vi "TruncI64.vi"(5 "Decimal places":i8, 6 "Number":i64) -> (2 "Truncated number":i64)   [LabVIEW 2017, in "GPNumeric.lvlib"]
doc: "Truncates <B>Number</B> to a number of <B>Decimal places</B>.\n\nSet <B>Decimal places</B> to a negative number to truncate to nearest 10, nearest 100 and so on. E.g. to truncate 782 to the nearest hundred, you set <B>Decimal places</B> to -2 and the <B>Truncated number</B> will be 700.\n\nThis VI is inlined.\n\nSteen Schmidt\nGPower\n16/5 2014"
uses:
  GPNumeric.lvlib
panel:
  # "Copyright © 2014\nGPower\nSee enclosed license file for terms and conditions"
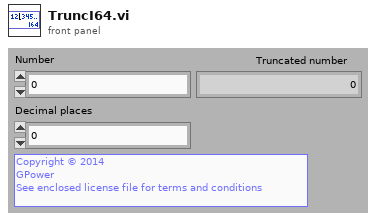
[diagram p1: front panel]
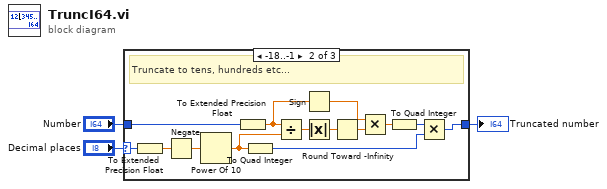
[diagram p0: block diagram]
diagram:
  n1 = case shown="-18..-1" "Decimal places" {
    selector: "Decimal places" -> [_ w14 _]
    tunnel: [_ w11 w18] -> w3
    tunnel: "Number" -> [_ w12 w18]
    frame ..-19 {
      # "Truncate above max value; Return zero."
    }
    frame -18..-1 {
      # "Truncate to tens, hundreds etc..."
      n2 = To Extended Precision Float(1:w14) -> (0:w13:ext)
      n3 = Negate(x=w13) -> (-x=w17:ext)
      n4 = Power Of 10(x=w17) -> (10^x=w10:ext)
      n5 = To Extended Precision Float(1:w12) -> (0:w5:ext)
      n6 = To Quad Integer(1:w10) -> (0:w16:i64)
      n7 = Divide(x=w5, y=w10) -> (x/y=w4:ext)
      n8 = Sign(1:w5) -> (0:w6:ext)
      n9 = Absolute Value(x=w4) -> (abs(x)=w9:ext)
      n10 = Round Toward -Infinity(1:w9) -> (0:w8:ext)
      n11 = Multiply(x=w6, y=w8) -> (x*y=w7:ext)
      n12 = To Quad Integer(1:w7) -> (0:w15:i64)
      n13 = Multiply(x=w15, y=w16) -> (x*y=w11:i64)
    }
    frame 0.. {
      # "Truncate to n decimal places; return integer unchanged."
    }
  }
  "Truncated number" <- w3
